vi "config parameter save.vi"(7 "ctl":T2(ring), 8 "error in":errorcluster caption="에러 입력(에러 없음)") -> (0 "error out":errorcluster caption="에러 출력", 2 "open cancelled":bool caption="취소됨", 3 "Config Parameter 2":T1 {"Acceleration Condition"."Filter cutoff freq" max=100; "Acceleration Condition"."Shock duration pecent [%]" max=100 format="%#.0f"})   [LabVIEW 2016]
uses:
  <vilib>/Utility/xml.llb/Write to XML File(string).vi
  <vilib>/Utility/xml.llb/Read From XML File(string).vi
panel:
  # "Select    Ch.    Initial"
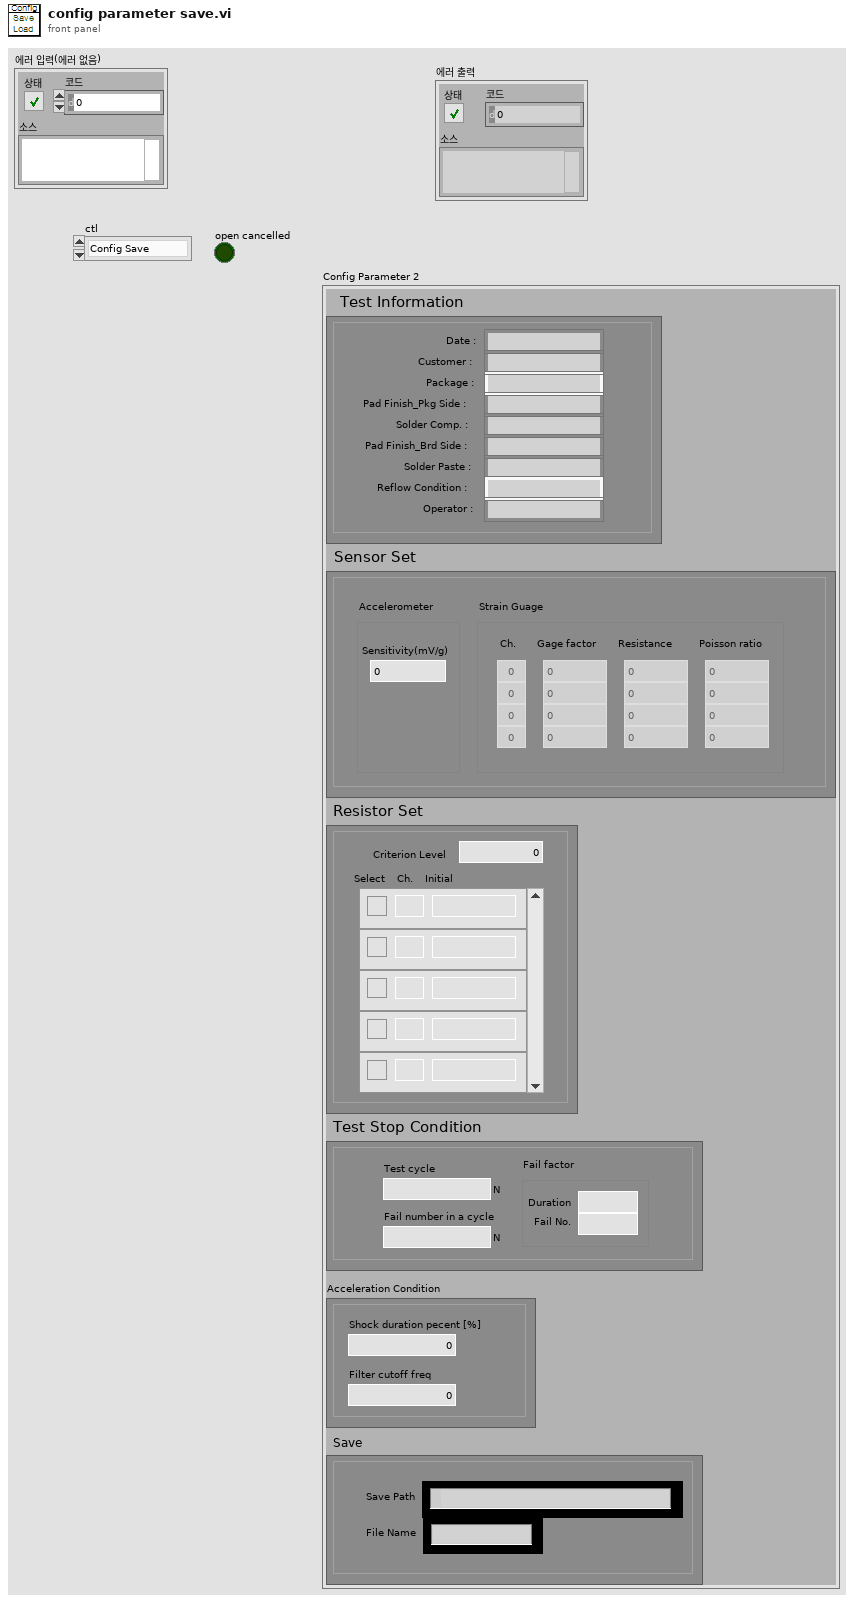
[diagram p1: front panel]
types:
  T1 = cluster{"Test Information":cluster{"date":string, "custom":string, "oper":string, "package":string, "pkg side":string, "solder":string, "brd side":string, "paste":string, "reflow":string}, "Sensor Set":cluster{"Accelerometer":cluster{"Sensitivity(mV/g)":dbl}, "Strain Guage":cluster{"Ch.":dbl[], "Gage factor":dbl[], "Resistance":dbl[], "Poisson ratio":dbl[]}}, "Resistor Set":cluster{"Criterion Level":dbl, "Res. Set":cluster{"Res. Ch":dbl, "Res. Active":bool, "Res Initial":dbl}[]}, "Test Stop Condition":cluster{"Test cycle":u16, "Fail number in a cycle":u16, "Fail factor":cluster{"Duration":u16, "Fail No.":u16}}, "Acceleration Condition":cluster{"Shock duration pecent [%]":u16, "Filter cutoff freq":u32}, "Save":cluster{"Save Path":path, "File Name":string}}
  T2 = enum16{"Config Save", "Config Load", "LastRUN Save", "LastRUN Load"}
  T3 = cluster{"Test Information":cluster{"date":string, "custom":string, "oper":string, "package":string, "pkg side":string, "solder":string, "brd side":string, "paste":string, "reflow":string}, "Sensor Set":cluster{"Accelerometer":cluster{"Sensitivity(mV/g)":dbl}, "Strain Guage":cluster{"Ch.":dbl[], "Gage factor":dbl[], "Resistance":dbl[], "Poisson ratio":dbl[]}}, "Resistor Set":cluster{"Criterion Level":dbl, "Res. Set":cluster{"Res. Ch":dbl, "Res. Active":bool, "Res Initial":dbl}[]}, "Test Stop Condition":cluster{"Test cycle":u16, "Fail number in a cycle":u16, "Fail factor":cluster{"Duration":u16, "Fail No.":u16}}, "Acceleration Condition ":cluster{"Shock duration pecent [%]":u16, "Filter cutoff freq":u32}, "Save":cluster{"Save Path":path, "File Name":string}}
  T4 = enum16{"open", "replace", "create", "open or create", "replace or create", "replace or create with confirmation"}
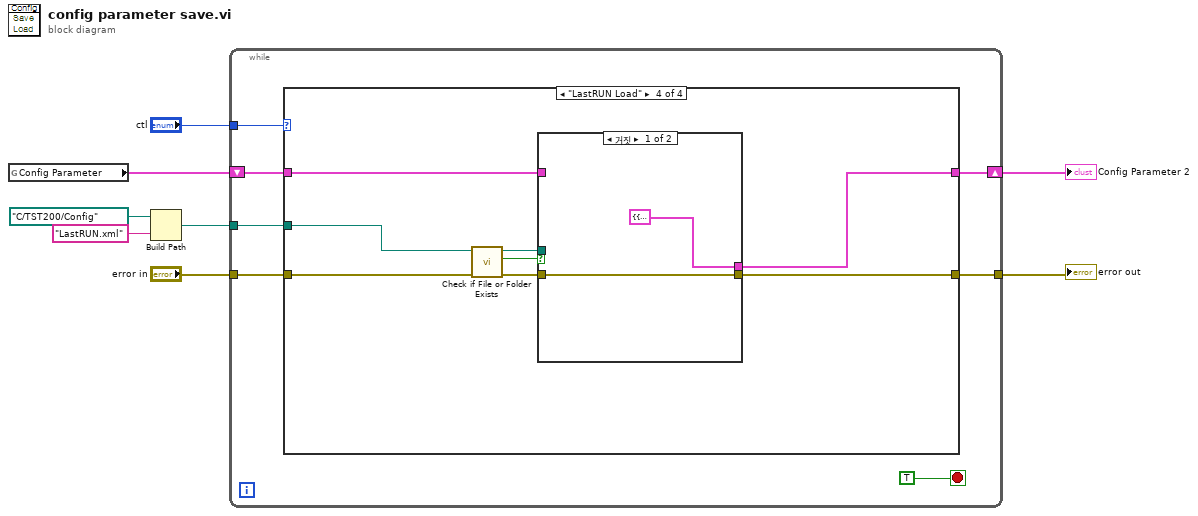
[diagram p0: block diagram]
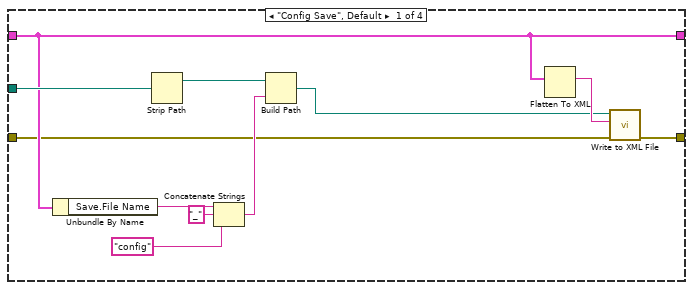
[diagram p2: hidden frame]
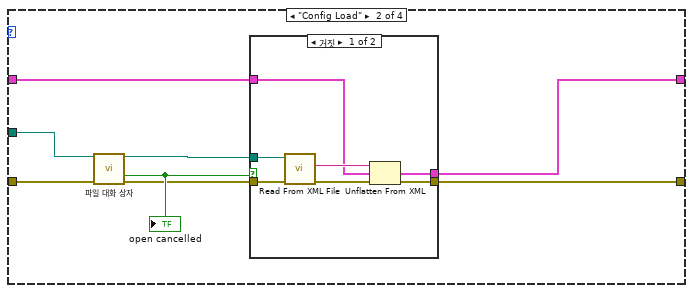
[diagram p3: hidden frame]
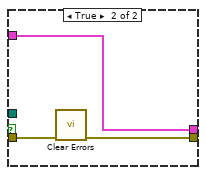
[diagram p4: hidden frame]
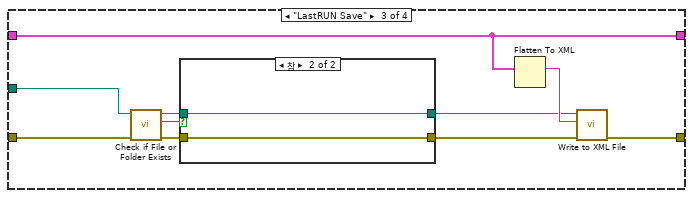
[diagram p5: hidden frame]
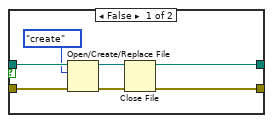
[diagram p6: hidden frame]
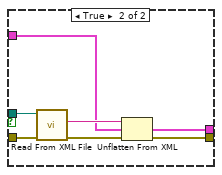
[diagram p7: hidden frame]
diagram:
  n1 = global read "글로벌_Config Parameter.vi" "Config Parameter"() -> (w1:T3)
  n2 = Build Path(base path=path "C:/TST200/Config" ("XML File Path"), name or relative path="LastRUN.xml" ("이름 또는 상대 경로")) -> (appended path=w3:path)
  n3 = while {
    tunnel: "error in" -> [w15]
    tunnel: [w14] -> w7
    tunnel: "ctl" -> [w13]
    tunnel: w3 -> [w11]
    shift-right: [w10] -> w2
    shift-left: w1 -> [w12]
    stop <- TRUE stop-if-true
    n4 = case shown="\"LastRUN Load\"" w13 {
      tunnel: w12 -> [w20 w31 w47 w71]
      tunnel: w11 -> [w23 w34 w46 w64]
      tunnel: w15 -> [w17 w29 w49 w68]
      tunnel: [w24 w28 w48 w69] -> w14
      tunnel: [w20 w27 w47 w70] -> w10
      frame "Config Save", Default {
        n5 = Unbundle By Name(w20) -> ("Save.File Name"=w26:string)
        n6 = Strip Path(path=w23) -> (stripped path=w22:path)  [unwired: 1 out]
        n7 = Concatenate Strings(w26, "_" ("문자열"), "config" ("문자열")) -> (w21:string)
        n8 = Build Path(base path=w22, name or relative path=w21) -> (appended path=w16:path)
        n9 = Flatten To XML(anything=w20) -> (xml string=w25:string)
        n10 = call-poly <vilib>:"Write to XML File.vi"("error in (no error)"=w17, "XML Input"=w25, "XML File Path"=w16) -> ("error out"=w24:errorcluster)  [unwired: 6 in, 2 out]
      }
      frame "Config Load" {
        n11 = call "파일 대화 상자"("start path"=w34, "error in"=w29) -> ("selected path"=w32:path, "cancelled"=w33:bool, "error out"=w30:errorcluster)  [unwired: 10 in, 1 out]
        "open cancelled" <- w33
        n12 = case shown="거짓" w33 {
          tunnel: w32 -> [w40 _]
          tunnel: w31 -> [w39 w44]
          tunnel: [w38 w44] -> w27
          tunnel: w30 -> [w36 w43]
          tunnel: [w35 w42] -> w28
          frame False {
            n13 = call-poly <vilib>:"Read From XML File.vi"("error in (no error)"=w36, "XML File Path"=w40) -> ("error out"=w37:errorcluster, "XML Elements"=w41:string)  [unwired: 7 in, 1 out]
            n14 = Unflatten From XML(xml string=w41, type=w39, error in (no error)=w37) -> (value=w38:T3, error out=w35:errorcluster)
          }
          frame True {
            n15 = call <vilib>:"Clear Errors.vi"("error in (no error)"=w43) -> ("error out"=w42:errorcluster)  [unwired: 5 in, 1 out]
          }
        }
      }
      frame "LastRUN Save" {
        n16 = call <vilib>:"Check if File or Folder Exists.vi"("error in (no error)"=w49, "path"=w46) -> ("error out"=w53:errorcluster, "file or folder exists?"=w51:bool, "dup path"=w52:path)  [unwired: 7 in]
        n17 = case shown="참" w51 {
          tunnel: w53 -> [w61 w63]
          tunnel: w52 -> [w60 w62]
          tunnel: [w55 w63] -> w50
          tunnel: [w56 w62] -> w45
          frame False {
            n18 = Open/Create/Replace File(file path (use dialog)=w60, error in=w61, operation (0:open)=T4."create" ("동작(0:open)")) -> (refnum out=w57:refnum<file>, error out=w58:errorcluster)  [unwired: 3 in, 1 out]
            n19 = Close File(refnum=w57, error in=w58) -> (path=w56:path, error out=w55:errorcluster)
          }
          frame True {
          }
        }
        n20 = Flatten To XML(anything=w47) -> (xml string=w54:string)
        n21 = call-poly <vilib>:"Write to XML File.vi"("error in (no error)"=w50, "XML Input"=w54, "XML File Path"=w45) -> ("error out"=w48:errorcluster)  [unwired: 6 in, 2 out]
      }
      frame "LastRUN Load" {
        n22 = call <vilib>:"Check if File or Folder Exists.vi"("error in (no error)"=w68, "path"=w64) -> ("error out"=w65:errorcluster, "file or folder exists?"=w66:bool, "dup path"=w67:path)  [unwired: 7 in]
        n23 = case shown="거짓" w66 {
          tunnel: w71 -> [_ w79]
          tunnel: [T3 {"Test Information"={"date"="", "custom"="", "oper"="", "package"="", "pkg side"="", "solder"="", "brd side"="", "paste"="", "reflow"=""}, "Sensor Set"={"Accelerometer"={"Sensitivity(mV/g)"=0.0}, "Strain Guage"={"Ch."=[], "Gage factor"=[], "Resistance"=[], "Poisson ratio"=[]}}, "Resistor Set"={"Criterion Level"=0.0, "Res. Set"=[]}, "Test Stop Condition"={"Test cycle"=0, "Fail number in a cycle"=0, "Fail factor"={"Duration"=0, "Fail No."=0}}, "Acceleration Condition "={"Shock duration pecent [%]"=0, "Filter cutoff freq"=0}, "Save"={"Save Path"=path "", "File Name"=""}} ("Config Parameter") w78] -> w70
          tunnel: [w73 w76] -> w69
          tunnel: w67 -> [_ w75]
          tunnel: w65 -> [w73 w74]
          frame False {
          }
          frame True {
            n24 = call-poly <vilib>:"Read From XML File.vi"("error in (no error)"=w74, "XML File Path"=w75) -> ("error out"=w77:errorcluster, "XML Elements"=w80:string)  [unwired: 7 in, 1 out]
            n25 = Unflatten From XML(xml string=w80, type=w79, error in (no error)=w77) -> (value=w78:T3, error out=w76:errorcluster)
          }
        }
      }
    }
  }
  "error out" <- w7
  "Config Parameter 2" <- w2
